vi "Close Shared Variables.vi"(8 "error in (no error)":errorcluster, 11 "Shared Variable Cluster":T1) -> (0 "error out":errorcluster)   [LabVIEW 2012, in "Shared Variable Custom Device.lvlib"]
uses:
  Shared Variable Custom Device.lvlib
  Shared Variable/Shared Variable Cluster.ctl
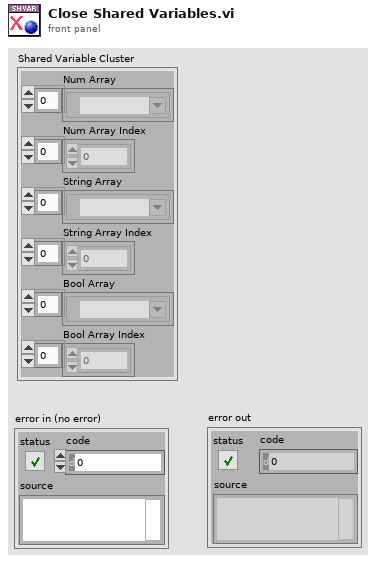
[diagram p1: front panel]
types:
  T1 = typedef "Shared Variable Custom Device.lvlib/Shared Variable Cluster.ctl" = cluster{"Num Array":refnum<k21>[], "Num Array Index":i32[], "String Array":refnum<k21>[], "String Array Index":i32[], "Bool Array":refnum<k21>[], "Bool Array Index":i32[]}
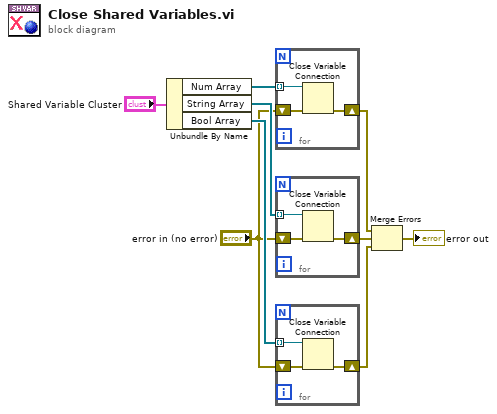
[diagram p0: block diagram]
diagram:
  n1 = Unbundle By Name("Shared Variable Cluster") -> ("Num Array"=w9:refnum<k21>[], "String Array"=w7:refnum<k21>[], "Bool Array"=w6:refnum<k21>[])
  n2 = for {
    tunnel: w9 -> [w12] mode=indexing
    shift-right: [w10] -> w4
    shift-left: "error in (no error)" -> [w11]
    n3 = Close Variable Connection(8:w11, 11:w12) -> (0:w10:errorcluster)
  }
  n4 = for {
    tunnel: w7 -> [w15] mode=indexing
    shift-right: [w13] -> w3
    shift-left: "error in (no error)" -> [w14]
    n5 = Close Variable Connection(8:w14, 11:w15) -> (0:w13:errorcluster)
  }
  n6 = for {
    tunnel: w6 -> [w18] mode=indexing
    shift-right: [w16] -> w2
    shift-left: "error in (no error)" -> [w17]
    n7 = Close Variable Connection(8:w17, 11:w18) -> (0:w16:errorcluster)
  }
  n8 = Merge Errors(w4, w3, w2) -> (→"error out":errorcluster)
